vi "System Explorer - Copy PPLTemplates for System Explorer.vi"(7 "CD Name":string, 8 "error in (no error)":errorcluster, 10 "CD Template":refnum<class "NIVS_CD Template.lvclass">, 11 "System Explorer folder":path) -> (0 "error out":errorcluster)   [LabVIEW 2020, in "NIVS_Consolidated_CDW_MetaDataObj.lvclass"]
doc: "Copy the templates for the System Explorer library into the System Explorer folder and disconnect the templates from the owning library."
uses:
  NIVS_Consolidated_CDW_MetaDataObj.lvclass
  Template Classes/NIVS_CD Template/NIVS_CD Template.lvclass
  CD System Explorer lvlib.ctl
  CD Shared lvlib.ctl
  Common.ctl
  Template Classes/NIVS_CD Template/NIVS_CD Template.lvclass/NIVS_CD Template.ctl
  Template Classes/NIVS_CD Template/Read Support Runtime Configuration.vi
  CD System Explorer lvlib.vi
  CD Shared lvlib.vi
  Common.vi
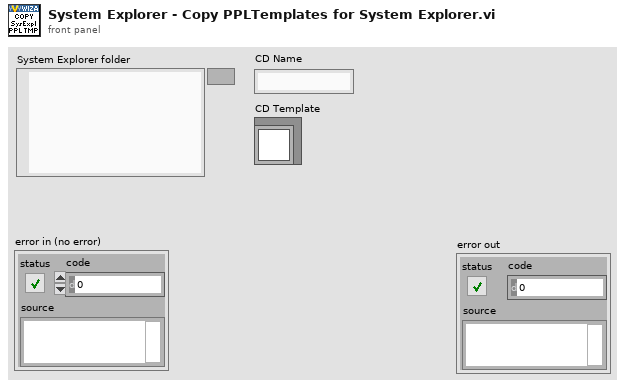
[diagram p1: front panel]
types:
  T1 = typedef "NIVS_Consolidated_CDW_MetaDataObj.lvclass/CD System Explorer lvlib.ctl" = enum16{"LibraryFileName", "LibraryFolderName", "System Explorer.FolderName", "System Explorer.Dynamically Called.FolderName", "System Explorer.Dynamically Called.Extra Pages.FolderName", "System Explorer.Dynamically Called.Extra Pages.TemplatePathAndName", "System Explorer.Dynamically Called.Main Page.VIName", "System Explorer.Dynamically Called.Main Page.TemplatePathAndName", "System Explorer.Dynamically Called.Initialization VI.VIName", "System Explorer.Dynamically Called.Initialization VI.TemplatePathAndName", "System Explorer.SubVI.FolderName", "System Explorer.Types.FolderName", "System Explorer.ActionVIOnCompile.VIName", "System Explorer.ActionVIOnRecompile.VIName", "System Explorer.ExportConfigRTM.VIName", "System Explorer.PPL.ExportConfigRTM.VIName", "System Explorer.LoadHelpFile.VIName", "System Explorer.PPL.LoadHelpFile.VIName", "System Explorer.SetRTDriverVIsFilePaths.VIName", "System Explorer.ClearRTDriverVIs.VIName"}
  T2 = typedef "NIVS_Consolidated_CDW_MetaDataObj.lvclass/Common.ctl" = enum16{"ProjectName", "TemplatesFolderName", "PPLTemplatesFolderName", "ProjectTemplatePathAndName", "ProjectPPLTemplatePathAndName", "TimingAndSyncFolderName", "CustomDeviceFolderName", "PathToTemplates", "PathToPPLTemplates", "PathToExplorerPPLTemplates", "PathToEnginePPLTemplates", "PathToConfigurationFile", "ProjectConfigurationName"}
  T3 = typedef "NIVS_Consolidated_CDW_MetaDataObj.lvclass/CD Shared lvlib.ctl" = enum16{"LibraryFileName", "LibraryFolderName", "ConstantsVI.VIPathAndName", "Shared.FolderName", "Shared.Types.FolderName", "Shared.Constants.VIName", "Shared.Constants.VITemplateName", "Shared.Constants.VITemplatePathAndName", "Shared.CompiledSettings.RelativePath", "Shared.Constants.RelativePath", "Shared.CompiledSettings.Name", "Shared.CompiledSettings.Name.NoExtension", "Shared.CompiledSettings.ClusterName"}
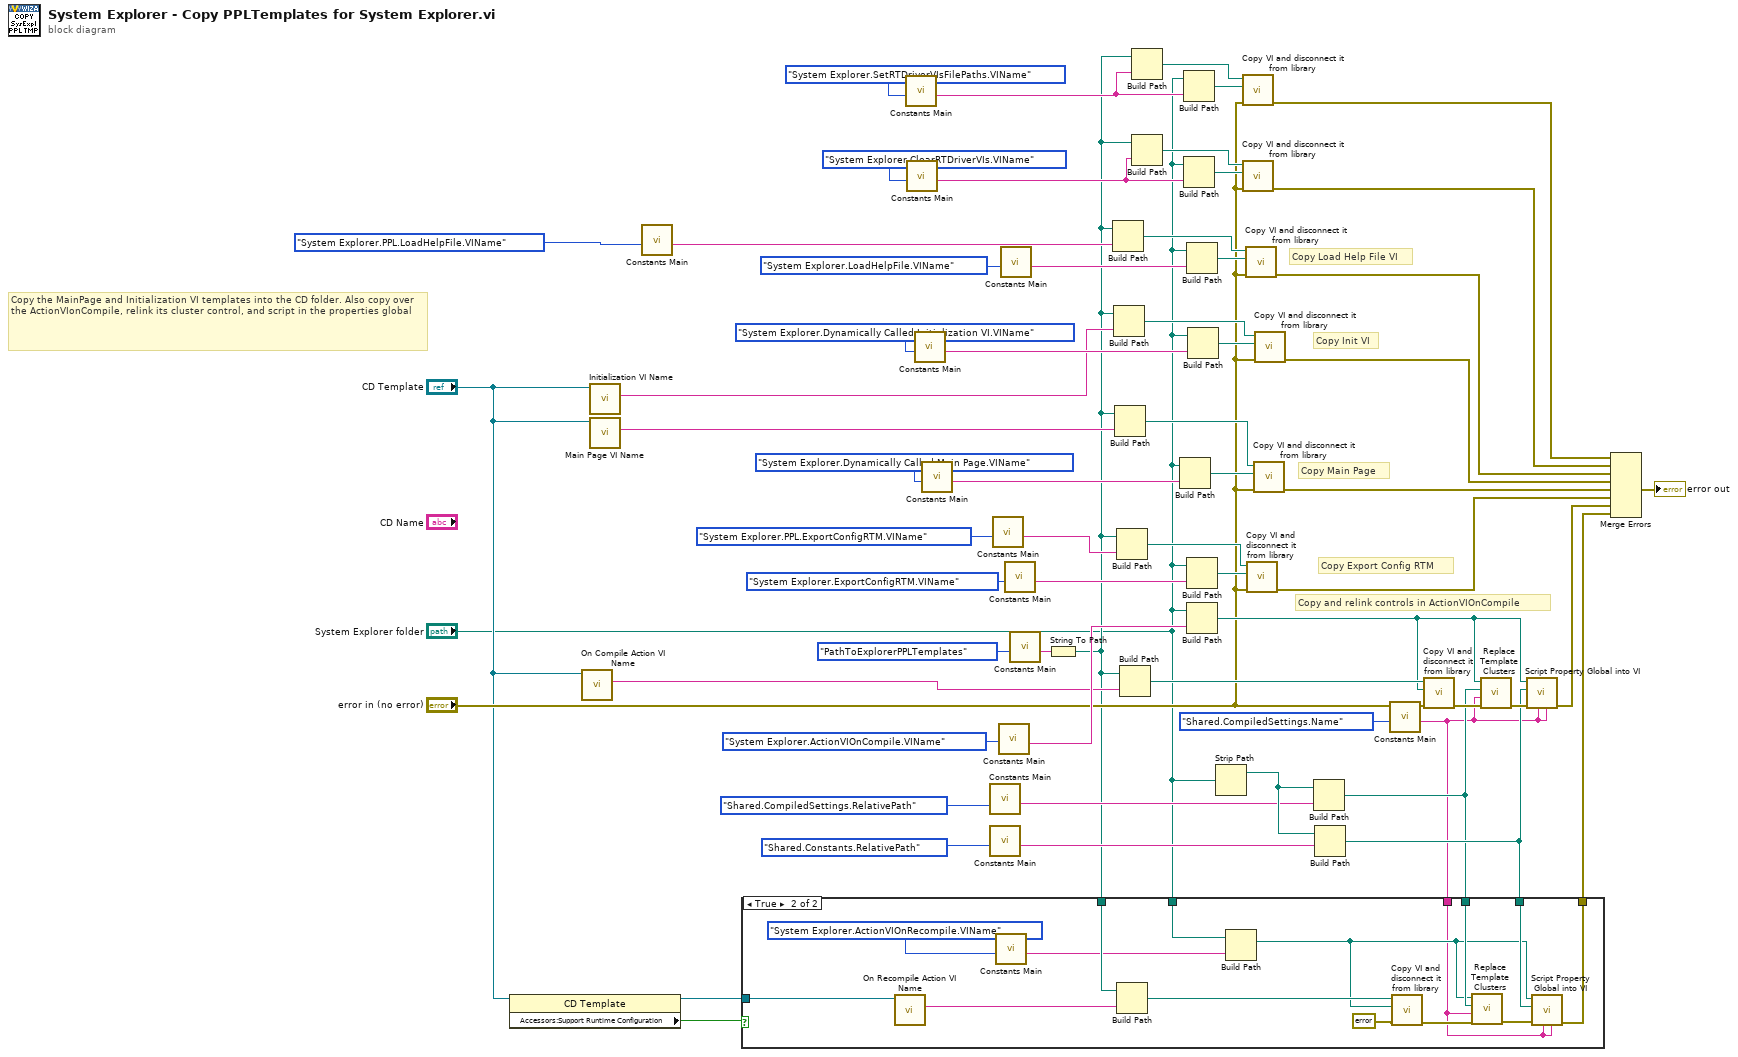
[diagram p0: block diagram]
diagram:
  # "Copy Load Help File VI"
  # "Copy the MainPage and Initialization VI templates into the CD folder. Also copy over the ActionVIonCompile, relink its cluster control, and script in the properties global"
  # "Copy Export Config RTM"
  # "Copy and relink controls in ActionVIOnCompile"
  # "Copy Main Page"
  # "Copy Init VI"
  n1 = property class="CD Template"(reference="CD Template") -> (reference out=w8:refnum<class "NIVS_CD Template.lvclass">, "Accessors:Support Runtime Configuration"=w5:bool)  [unwired: 1 in, 1 out]
  n2 = call-dynamic "On Compile Action VI Name.vi"("CD Template in"="CD Template") -> ("On Compile Action VI Name"=w28:string)  [unwired: 10 in]
  n3 = call-dynamic "Initialization VI Name.vi"("CD Template in"="CD Template") -> ("Initialization VI Name"=w30:string)  [unwired: 10 in]
  n4 = call-dynamic "Main Page VI Name.vi"("CD Template in"="CD Template") -> ("Main Page VI Name"=w29:string)  [unwired: 10 in]
  n5 = call-poly "Constants Main.vi"("Action"=CD_System_Explorer_lvlib."System Explorer.PPL.LoadHelpFile.VIName") -> ("Output"=w12:string)  [unwired: 10 in]
  n6 = call-poly "Constants Main.vi"("Action"=CD_System_Explorer_lvlib."System Explorer.SetRTDriverVIsFilePaths.VIName") -> ("Output"=w16:string)  [unwired: 10 in]
  n7 = call-poly "Constants Main.vi"("Action"=CD_System_Explorer_lvlib."System Explorer.ClearRTDriverVIs.VIName") -> ("Output"=w24:string)  [unwired: 10 in]
  n8 = call-poly "Constants Main.vi"("Action"=CD_System_Explorer_lvlib."System Explorer.Dynamically Called.Initialization VI.VIName") -> ("Output"=w53:string)  [unwired: 10 in]
  n9 = call-poly "Constants Main.vi"("Action"=CD_System_Explorer_lvlib."System Explorer.Dynamically Called.Main Page.VIName") -> ("Output"=w52:string)  [unwired: 10 in]
  n10 = call-poly "Constants Main.vi"("Action"=CD_Shared_lvlib."Shared.CompiledSettings.RelativePath") -> ("Output"=w26:string)  [unwired: 10 in]
  n11 = call-poly "Constants Main.vi"("Action"=CD_Shared_lvlib."Shared.Constants.RelativePath") -> ("Output"=w45:string)  [unwired: 10 in]
  n12 = call-poly "Constants Main.vi"("Action"=CD_System_Explorer_lvlib."System Explorer.PPL.ExportConfigRTM.VIName") -> ("Output"=w10:string)  [unwired: 10 in]
  n13 = call-poly "Constants Main.vi"("Action"=CD_System_Explorer_lvlib."System Explorer.ActionVIOnCompile.VIName") -> ("Output"=w47:string)  [unwired: 10 in]
  n14 = call-poly "Constants Main.vi"("Action"=CD_System_Explorer_lvlib."System Explorer.LoadHelpFile.VIName") -> ("Output"=w35:string)  [unwired: 10 in]
  n15 = call-poly "Constants Main.vi"("Action"=CD_System_Explorer_lvlib."System Explorer.ExportConfigRTM.VIName") -> ("Output"=w40:string)  [unwired: 10 in]
  n16 = call-poly "Constants Main.vi"("Action"=Common."PathToExplorerPPLTemplates") -> ("Output"=w58:string)  [unwired: 10 in]
  n17 = String To Path(string=w58) -> (path=w7:path)
  n18 = Build Path(base path=w7, name or relative path=w12) -> (appended path=w34:path)
  n19 = Build Path(base path=w7, name or relative path=w30) -> (appended path=w54:path)
  n20 = Build Path(base path=w7, name or relative path=w29) -> (appended path=w55:path)
  n21 = Build Path(base path=w7, name or relative path=w10) -> (appended path=w43:path)
  n22 = Build Path(base path=w7, name or relative path=w28) -> (appended path=w57:path)
  n23 = Build Path(base path=w7, name or relative path=w16) -> (appended path=w20:path)
  n24 = Build Path(base path=w7, name or relative path=w24) -> (appended path=w23:path)
  n25 = Build Path(base path="System Explorer folder", name or relative path=w52) -> (appended path=w36:path)
  n26 = Build Path(base path="System Explorer folder", name or relative path=w16) -> (appended path=w21:path)
  n27 = Build Path(base path="System Explorer folder", name or relative path=w24) -> (appended path=w22:path)
  n28 = Build Path(base path="System Explorer folder", name or relative path=w35) -> (appended path=w33:path)
  n29 = Build Path(base path="System Explorer folder", name or relative path=w40) -> (appended path=w42:path)
  n30 = Build Path(base path="System Explorer folder", name or relative path=w47) -> (appended path=w50:path)
  n31 = Build Path(base path="System Explorer folder", name or relative path=w53) -> (appended path=w60:path)
  n32 = Strip Path(path="System Explorer folder") -> (stripped path=w49:path)  [unwired: 1 out]
  n33 = call "Copy VI and disconnect it from library.vi"("error in (no error)"="error in (no error)", "VI Target Path"=w21, "VI Source Path"=w20) -> ("error out"=w18:errorcluster)  [unwired: 8 in]
  n34 = call "Copy VI and disconnect it from library.vi"("error in (no error)"="error in (no error)", "VI Target Path"=w22, "VI Source Path"=w23) -> ("error out"=w19:errorcluster)  [unwired: 8 in]
  n35 = call "Copy VI and disconnect it from library.vi"("error in (no error)"="error in (no error)", "VI Target Path"=w33, "VI Source Path"=w34) -> ("error out"=w31:errorcluster)  [unwired: 8 in]
  n36 = call "Copy VI and disconnect it from library.vi"("error in (no error)"="error in (no error)", "VI Target Path"=w42, "VI Source Path"=w43) -> ("error out"=w38:errorcluster)  [unwired: 8 in]
  n37 = call "Copy VI and disconnect it from library.vi"("error in (no error)"="error in (no error)", "VI Target Path"=w36, "VI Source Path"=w55) -> ("error out"=w37:errorcluster)  [unwired: 8 in]
  n38 = call "Copy VI and disconnect it from library.vi"("error in (no error)"="error in (no error)", "VI Target Path"=w60, "VI Source Path"=w54) -> ("error out"=w59:errorcluster)  [unwired: 8 in]
  n39 = Build Path(base path=w49, name or relative path=w26) -> (appended path=w3:path)
  n40 = Build Path(base path=w49, name or relative path=w45) -> (appended path=w4:path)
  n41 = call-poly "Constants Main.vi"("Action"=CD_Shared_lvlib."Shared.CompiledSettings.Name") -> ("Output"=w1:string)  [unwired: 10 in]
  n42 = case shown="True" w5 {
    tunnel: w8 -> [_ w78]
    tunnel: w7 -> [_ w77]
    tunnel: "System Explorer folder" -> [_ w75]
    tunnel: w4 -> [_ w72]
    tunnel: w3 -> [_ w71]
    tunnel: [_ w66] -> w2
    tunnel: w1 -> [_ w64]
    frame False {
    }
    frame True {
      n43 = call-dynamic "On Recompile Action VI Name.vi"("CD Template in"=w78) -> ("On Recompile Action VI Name"=w76:string)  [unwired: 10 in]
      n44 = call-poly "Constants Main.vi"("Action"=CD_System_Explorer_lvlib."System Explorer.ActionVIOnRecompile.VIName") -> ("Output"=w73:string)  [unwired: 10 in]
      n45 = Build Path(base path=w77, name or relative path=w76) -> (appended path=w70:path)
      n46 = Build Path(base path=w75, name or relative path=w73) -> (appended path=w69:path)
      n47 = call "Copy VI and disconnect it from library.vi"("error in (no error)"=errorcluster {"status"=FALSE, "code"=0, "source"=""}, "VI Target Path"=w69, "VI Source Path"=w70) -> ("error out"=w68:errorcluster)  [unwired: 8 in]
      n48 = call "Replace Template Clusters.vi"("error in (no error)"=w68, "Control Name"=w64, "Path to Cluster to Replace"=w71, "Path to VI"=w69) -> ("error out"=w67:errorcluster)  [unwired: 7 in]
      n49 = call "Script Property Global into VI.vi"("GlobalControlName"=w64, "StringConstantToReplace"=w64, "error in (no error)"=w67, "Path to Global"=w72, "Path to VI"=w69) -> ("error out"=w66:errorcluster)  [unwired: 6 in]
    }
  }
  n50 = call "Copy VI and disconnect it from library.vi"("error in (no error)"="error in (no error)", "VI Target Path"=w50, "VI Source Path"=w57) -> ("error out"=w56:errorcluster)  [unwired: 8 in]
  n51 = call "Replace Template Clusters.vi"("error in (no error)"=w56, "Control Name"=w1, "Path to Cluster to Replace"=w3, "Path to VI"=w50) -> ("error out"=w51:errorcluster)  [unwired: 7 in]
  n52 = call "Script Property Global into VI.vi"("GlobalControlName"=w1, "StringConstantToReplace"=w1, "error in (no error)"=w51, "Path to Global"=w4, "Path to VI"=w50) -> ("error out"=w39:errorcluster)  [unwired: 6 in]
  n53 = Merge Errors(w18, w19, w31, w59, w37, w38, w39, w2) -> (→"error out":errorcluster)
